vi "Read State.vi"(8 "error in (no error)":errorcluster, 11 "TwinCAT ADS in":refnum<class "TwinCAT ADS.lvclass">) -> (0 "error out":errorcluster, 1 "State Information":T1, 3 "TwinCAT ADS out":refnum<class "TwinCAT ADS.lvclass">)   [LabVIEW 2018, in "TwinCAT ADS.lvclass"]
uses:
  TwinCAT ADS.lvclass
  Controls/State Information.ctl
  TwinCAT ADS.lvclass/TwinCAT ADS.ctl
  TwinCAT.Ads
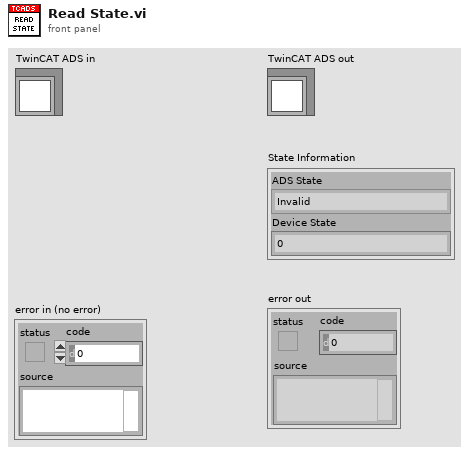
[diagram p1: front panel]
types:
  T1 = typedef "TwinCAT ADS.lvclass/State Information.ctl" = cluster{"ADS State":enum16{"Invalid", "Idle", "Reset", "Init", "Start", "Run", "Stop", "SaveConfig", "LoadConfig", "PowerFailure", "PowerGood", "Error", "Shutdown", "Suspend", "Resume", "Config", "Reconfig", "Stopping, Maxstates", "Incompatible", "Exception"}, "Device State":i16}
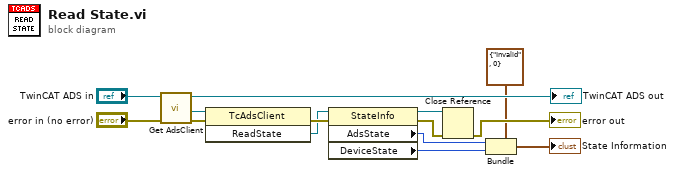
[diagram p0: block diagram]
diagram:
  n1 = call "Get AdsClient.vi"("error in (no error)"="error in (no error)", "TwinCAT ADS in"="TwinCAT ADS in") -> ("error out"=w5:errorcluster, ".NET TcAdsClient"=w4:refnum<k24>, "TwinCAT ADS out"=→"TwinCAT ADS out":refnum<class "TwinCAT ADS.lvclass">)  [unwired: 7 in]
  n2 = invoke class="TcAdsClient" method="ReadState"(reference=w4, error in=w5) -> (error out=w9:errorcluster, "ReadState"=w8:refnum<k24>)  [unwired: 1 in, 1 out]
  n3 = property class="StateInfo"(reference=w8, error in=w9) -> (reference out=w1:refnum<k24>, error out=w2:errorcluster, "AdsState"=w7:i16, "DeviceState"=w6:i16)
  n4 = Close Reference(reference=w1, error in (no error)=w2) -> (error out=→"error out":errorcluster)
  n5 = Bundle(cluster=T1 {"ADS State"=enum."Invalid", "Device State"=0} ("State Information"), "ADS State"=w7, "Device State"=w6) -> (→"State Information":T1)
